vi "WPI_CANJaguar_ScheduledPeriodicUpdates.vi"(8 "Fields In":T5[](array[typedef]), 9 "Update":bool, 10 "Status Channel Select":T6, 11 "CAN Jaguar Ref":T1={"DeviceStatus"={"status"=FALSE, "code"=0, "source"=""}, "Type"=enum."PWM", "PWM"={"PWM Channel"=enum."PWM 1", "DeadBand"={"Name"="", "maxPositivePwm"=0, "minPositivePwm"=0, "centerPwm"=0, "maxNegativePwm"=0, "minNegativePwm"=0, "angularRange"=0}}, "CAN"={"Device Number"=0, "SetOutput VI Ref"=variant(enum8{"Percent VBus", "Current", "Speed", "Position", "Voltage"} enum."Percent VBus"), "GetOutput VI Ref"=variant(refnum<k1> refnum), "Enable VI Ref"=variant(dbl 12.0), "Disable VI Ref"=variant(enum8{"Percent VBus", "Speed", "Position", "Slave", "Unchanged / Invalid", "Voltage Compensation", "Current", "Motion Profile"} enum."Percent VBus"), "Data"=variant}, "Invert"=FALSE}) -> (0 "Fields Out":T5[](array[typedef]))   [LabVIEW 2016]
uses:
  <vilib>/Rock Robotics/WPI/ThirdParty/CanMotor/CAN Jaguar/SubVIs/WPI_CANJaguar_StatusChannelSelect.ctl
  <vilib>/Rock Robotics/WPI/ThirdParty/CanMotor/CAN Jaguar/SubVIs/WPI_CAN_PeriodicStatusIDs.ctl
  <vilib>/Rock Robotics/WPI/MotorControl/WPI_MotorControlDeviceRef.ctl
  <vilib>/Rock Robotics/WPI/MotorControl/WPI_MotorControlType.ctl
  <vilib>/Rock Robotics/SystemInterfaces/DIO/FPGA_DIOPWMChannel.ctl
  <vilib>/Rock Robotics/WPI/PWM/WPI_PWMDeadband.ctl
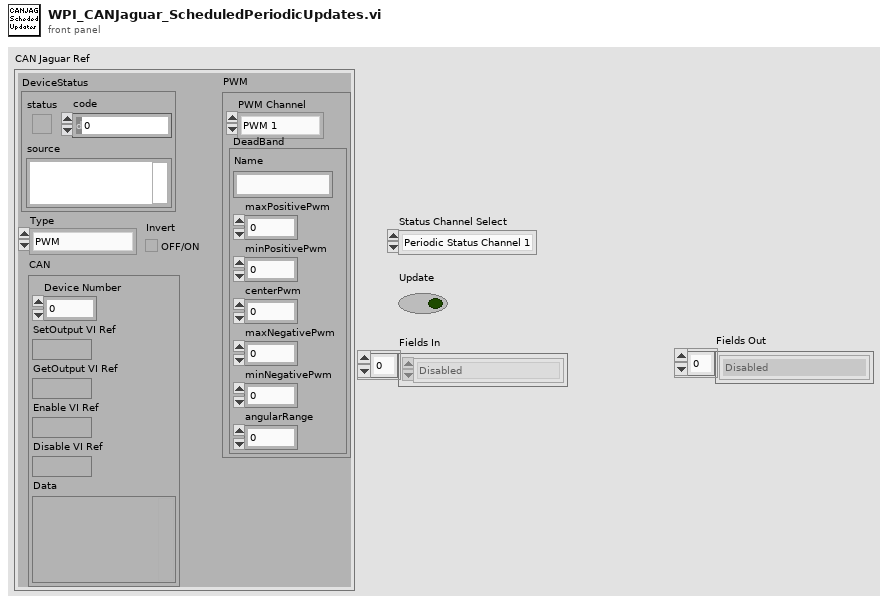
[diagram p1: front panel]
types:
  T1 = typedef "WPI_MotorControlDeviceRef.ctl" = cluster{"DeviceStatus":errorcluster, "Type":T2, "PWM":cluster{"PWM Channel":T3, "DeadBand":T4}, "CAN":cluster{"Device Number":u8, "SetOutput VI Ref":variant, "GetOutput VI Ref":variant, "Enable VI Ref":variant, "Disable VI Ref":variant, "Data":variant}, "Invert":bool}
  T2 = typedef "WPI_MotorControlType.ctl" = enum16{"PWM", "CAN"}
  T3 = typedef "FPGA_DIOPWMChannel.ctl" = enum8{"PWM 0", "PWM 1", "PWM 2", "PWM 3", "PWM 4", "PWM 5", "PWM 6", "PWM 7", "PWM 8", "PWM 9", "PWM MXP 0", "PWM MXP 1", "PWM MXP 2", "PWM MXP 3", "PWM MXP 4", "PWM MXP 5", "PWM MXP 6", "PWM MXP 7", "PWM MXP 8", "PWM MXP 9", "Invalid"}
  T4 = typedef "WPI_PWMDeadband.ctl" = cluster{"Name":string, "maxPositivePwm":i32, "minPositivePwm":i32, "centerPwm":i32, "maxNegativePwm":i32, "minNegativePwm":i32, "angularRange":u16}
  T5 = typedef "WPI_CAN_PeriodicStatusIDs.ctl" = enum16{"Disabled", "Percent VBus Out (Byte 0)", "Percent VBus Out (Byte 1)", "VBus (Byte 0)", "VBus (Byte 1)", "Current (Byte 0)", "Current (Byte 1)", "Temperature (Byte 0)", "Temperature (Byte 1)", "Position (Byte 0)", "Position (Byte 1)", "Position (Byte 2)", "Position (Byte 3)", "Speed (Byte 0)", "Speed (Byte 1)", "Speed (Byte 2)", "Speed (Byte 3)", "Limit Switches (No Clear)", "Limit Switches (Clear)", "Faults", "Sticky Faults (No Clear)", "Sticky Faults (Clear)", "Volts Out (Byte 0)", "Volts Out (Byte 1)", "Current Fault Counter", "Temperature Fault Counter", "VBus Fault Counter", "Gate Driver Fault Counter", "Comm Fault Counter", "CANSTS", "CANERR (Byte 0)", "CANERR (Byte 1)", "Power Cycle"}
  T6 = typedef "WPI_CANJaguar_StatusChannelSelect.ctl" = enum16{"Periodic Status Channel 1", "Periodic Status Channel 2", "Periodic Status Channel 3", "Periodic Status Channel 4", "On Demand Status"}
  T7 = cluster{"Device Number":u8, "Fields 0":T5[], "Fields 1":T5[], "Fields 2":T5[], "Fields 3":T5[]}[]
  T8 = cluster{"Device Number":u8, "Fields 0":T5[], "Fields 1":T5[], "Fields 2":T5[], "Fields 3":T5[]}
  T9 = cluster{"Device Number":u8, "Fields 0":T5[], "Fields 0":T5[], "Fields 0":T5[], "Fields 0":T5[]}
  T10 = cluster{"Device Number":u8, "Fields 0":T5[], "Fields 0":T5[], "Fields 0":T5[], "Fields 0":T5[]}[]
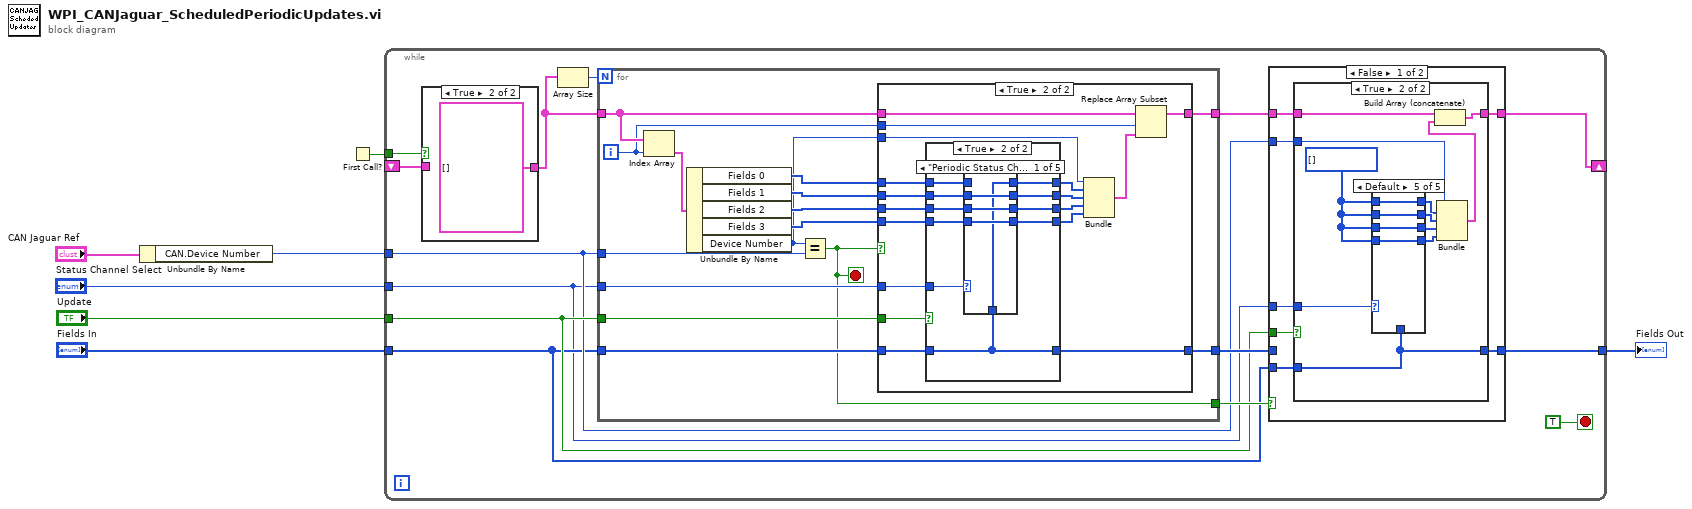
[diagram p0: block diagram]
diagram:
  n1 = Unbundle By Name("CAN Jaguar Ref") -> ("CAN.Device Number"=w1:u8)
  n2 = First Call?() -> (First Call?: T/F=w4:bool)
  n3 = while {
    tunnel: "Fields In" -> [w9]
    tunnel: "Update" -> [w11]
    tunnel: "Status Channel Select" -> [w8]
    tunnel: w4 -> [w20]
    tunnel: [w15] -> w3
    shift-right: [w13] -> _
    shift-left: _ -> [w19]
    tunnel: w1 -> [w10]
    stop <- TRUE stop-if-true
    n4 = case shown="True" w20 {
      tunnel: w19 -> [w156 _]
      tunnel: [w156 T7 []] -> w17
      frame False {
      }
      frame True {
      }
    }
    n5 = Array Size(array=w17) -> (size(s)=w18:i32)
    n6 = for {
      N: w18 -> [_]
      tunnel: w11 -> [w77]
      tunnel: w8 -> [w76]
      tunnel: [w67] -> w12
      tunnel: w17 -> [w66]
      tunnel: w10 -> [w68]
      tunnel: [w65] -> w16
      tunnel: w9 -> [w75]
      tunnel: [w74] -> w14
      i -> [w64]
      stop <- w65 stop-if-true
      n7 = Index Array(array=w66, index=w64) -> (element=w73:T8)
      n8 = Unbundle By Name(w73) -> ("Fields 0"=w72:T5[], "Fields 1"=w71:T5[], "Fields 2"=w70:T5[], "Fields 3"=w69:T5[], "Device Number"=w63:u8)
      n9 = Equal?(x=w63, y=w68) -> (x = y?=w65:bool)
      n10 = case shown="True" w65 {
        tunnel: w77 -> [_ w95]
        tunnel: w76 -> [_ w94]
        tunnel: w75 -> [_ w93]
        tunnel: [_ w92] -> w74
        tunnel: w72 -> [_ w91]
        tunnel: w71 -> [_ w90]
        tunnel: w70 -> [_ w89]
        tunnel: w69 -> [_ w88]
        tunnel: [w78 w86] -> w67
        tunnel: w66 -> [w78 w87]
        tunnel: w64 -> [_ w85]
        tunnel: w63 -> [_ w84]
        frame False {
        }
        frame True {
          n11 = case shown="True" w95 {
            tunnel: w94 -> [w105 w135]
            tunnel: w93 -> [_ w126]
            tunnel: [w103 w127] -> w82
            tunnel: w90 -> [w102 w132]
            tunnel: [w96 w126] -> w92
            tunnel: [w97 w130] -> w83
            tunnel: w91 -> [w104 w131]
            tunnel: [w101 w129] -> w81
            tunnel: w89 -> [w100 w133]
            tunnel: [w99 w128] -> w80
            tunnel: w88 -> [w98 w134]
            frame False {
              n12 = case shown="\"Periodic Status Channel 1\"" w105 {
                tunnel: w104 -> [w106 w111 w115 w119 w122]
                tunnel: [w109 w110 w117 w121 w125] -> w103
                tunnel: w102 -> [w109 w110 w117 w121 w125]
                tunnel: [w108 w113 w114 w120 w124] -> w101
                tunnel: w100 -> [w108 w113 w114 w120 w124]
                tunnel: [w107 w112 w116 w118 w123] -> w99
                tunnel: w98 -> [w107 w112 w116 w118 w123]
                tunnel: [w106 w111 w115 w119 w122] -> w97
                tunnel: [w106 w110 w114 w118 _] -> w96
                frame "Periodic Status Channel 1" {
                }
                frame "Periodic Status Channel 2" {
                }
                frame "Periodic Status Channel 3" {
                }
                frame "Periodic Status Channel 4" {
                }
                frame Default {
                }
              }
            }
            frame True {
              n13 = case shown="\"Periodic Status Channel 1\"" w135 {
                tunnel: w134 -> [w137 w141 w146 _ w153]
                tunnel: w133 -> [w138 w142 _ w149 w154]
                tunnel: w132 -> [w139 _ w145 w150 w152]
                tunnel: w131 -> [_ w143 w147 w151 w155]
                tunnel: [w136 w143 w147 w151 w155] -> w130
                tunnel: [w138 w142 w144 w149 w154] -> w129
                tunnel: [w137 w141 w146 w148 w153] -> w128
                tunnel: [w139 w140 w145 w150 w152] -> w127
                tunnel: w126 -> [w136 w140 w144 w148 _]
                frame "Periodic Status Channel 1" {
                }
                frame "Periodic Status Channel 2" {
                }
                frame "Periodic Status Channel 3" {
                }
                frame "Periodic Status Channel 4" {
                }
                frame Default {
                }
              }
            }
          }
          n14 = Bundle("Device Number"=w84, "Fields 0"=w83, "Fields 1"=w82, "Fields 2"=w81, "Fields 3"=w80) -> (w79:T8)  [unwired: 1 in]
          n15 = Replace Array Subset(array=w87, new element=w79, index=w85) -> (w86:T7)
        }
      }
    }
    n16 = case shown="False" w16 {
      tunnel: [w24 w62] -> w15
      tunnel: w14 -> [_ w62]
      tunnel: [w26 w61] -> w13
      tunnel: w12 -> [w27 w61]
      tunnel: w11 -> [w28 _]
      tunnel: w10 -> [w22 _]
      tunnel: w9 -> [w25 _]
      tunnel: w8 -> [w23 _]
      frame False {
        n17 = case shown="True" w28 {
          tunnel: w27 -> [w29 w40]
          tunnel: [w29 w39] -> w26
          tunnel: w25 -> [_ w36]
          tunnel: [_ w36] -> w24
          tunnel: w23 -> [_ w38]
          tunnel: w22 -> [_ w31]
          frame False {
          }
          frame True {
            w37 = T5[] [] items=["Disabled", "Percent VBus Out (Byte 0)", "Percent VBus Out (Byte 1)", "VBus (Byte 0)", "VBus (Byte 1)", "Current (Byte 0)", "Current (Byte 1)", "Temperature (Byte 0)", "Temperature (Byte 1)", "Position (Byte 0)", "Position (Byte 1)", "Position (Byte 2)", "Position (Byte 3)", "Speed (Byte 0)", "Speed (Byte 1)", "Speed (Byte 2)", "Speed (Byte 3)", "Limit Switches (No Clear)", "Limit Switches (Clear)", "Faults", "Sticky Faults (No Clear)", "Sticky Faults (Clear)", "Volts Out (Byte 0)", "Volts Out (Byte 1)", "Current Fault Counter", "Temperature Fault Counter", "VBus Fault Counter", "Gate Driver Fault Counter", "Comm Fault Counter", "CANSTS", "CANERR (Byte 0)", "CANERR (Byte 1)", "Power Cycle"] ("Fields 0")
            n18 = case shown="Default" w38 {
              tunnel: w37 -> [w42 w46 w51 _ w58]
              tunnel: w37 -> [w43 w47 _ w54 w59]
              tunnel: w37 -> [w44 _ w50 w55 w57]
              tunnel: w37 -> [_ w48 w52 w56 w60]
              tunnel: [w41 w48 w52 w56 w60] -> w32
              tunnel: [w43 w47 w49 w54 w59] -> w34
              tunnel: [w42 w46 w51 w53 w58] -> w35
              tunnel: [w44 w45 w50 w55 w57] -> w33
              tunnel: w36 -> [w41 w45 w49 w53 _]
              frame "Periodic Status Channel 1" {
              }
              frame "Periodic Status Channel 2" {
              }
              frame "Periodic Status Channel 3" {
              }
              frame "Periodic Status Channel 4" {
              }
              frame Default {
              }
            }
            n19 = Bundle("Device Number"=w31, "Fields 0"=w32, "Fields 0"=w33, "Fields 0"=w34, "Fields 0"=w35) -> (w30:T9)  [unwired: 1 in]
            n20 = Build Array (concatenate)(w40, w30) -> (w39:T10)
          }
        }
      }
      frame True {
      }
    }
  }
  "Fields Out" <- w3
